vi "barrierOrManMark.vi"(8 "error in (no error)":errorcluster, 9 "Number of Defenders\nWithout Duelist":i32, 10 "Game":refnum<class "Game.lvclass">, 11 "DefendAreaSkill in":refnum<class "DefendAreaSkill.lvclass">) -> (0 "error out":errorcluster, 1 "Enemy position\nto mark":dbl[](array[numeric]), 2 "Type of Defense Barrier":enum16{"Barreira", "Manmark"}(ring), 3 "DefendAreaSkill out":refnum<class "DefendAreaSkill.lvclass">)   [LabVIEW 2024, in "DefendAreaSkill.lvclass"]
uses:
  DefendAreaSkill.lvclass
  Game_class/Game.lvclass
  Team_class/OffensivePlay.ctl
  Game_class/Game.lvclass/Game.ctl
  Team_class/Team.lvclass/Team.ctl
  Events_class/Events.lvclass/Events.ctl
  Object_class/Object.lvclass/Object.ctl
  Object_class/Read x.vi
  Object_class/Read y.vi
  Team_class/Read RobotRef.vi
  Game_class/Read Utilities.lvclass.vi
  Game_class/Read EnemyRef.vi
  Game_class/Read Parameters.lvclass.vi
  Game_class/Read OffensiveTeam.vi
  Game_class/Read BallRef.vi
  Game_class/Read EventsRef.vi
  Events_class/Read id_enemy_ball_possesion.vi
  Team_class/Read OffensivePlay.vi
  Parameters_class/Read AttakingOurselves.vi
  Ally_class/Ally.lvclass
  C:/Users/ROBOIME2/Documents/SSL ROBOIME/SSL_AI/Team_class/Team.lvclass
  Enemy_class/Enemy.lvclass
  Robot_class/Robot.lvclass
  C:/Users/ROBOIME2/Documents/SSL ROBOIME/SSL_AI/Object_class/Object.lvclass
  Utilities_class/Utilities.lvclass
  Parameters_class/Parameters.lvclass
  Ball_class/Ball.lvclass
  Events_class/Events.lvclass
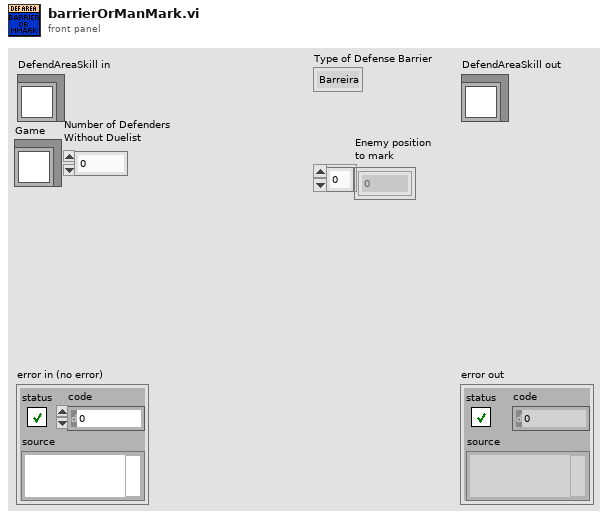
[diagram p1: front panel]
types:
  T1 = typedef "OffensivePlay.ctl" = enum16{"5RobotsPassGamePlay", "5PreparePassGame", "5RobotsKeeperGame", "KeeperPassToStriker", "5RobotsNormalGamePlay", "PrepareKeeperPass", "ACBPass", "ABCPass", "PrepareTriplePass", "TableWithStriker", "TableWith2ndStrikerPlay", "PrepareDoublePass", "PrepareRollToPass", "SimplePass", "PreparePass", "PassToStriker", "BallOutOfField", "PassTo2ndStriker", "StopOffensive", "Prepare Penalty Enemy", "EnemyPossessionAtEnemyField", "EnemyPossesionAtOurField", "TestPlay", "PreparePenaltyAlly", "KickPenaltyAlly", "PrepareKickoffAlly", "PrepareKickoffEnemy", "IndirectEnemy", "DirectEnemy", "PreparePassInGame1", "NormalGame", "DirectKick", "Pass", "Halt", "Timeout", "PassPlay", "PenaltyEnemy"}
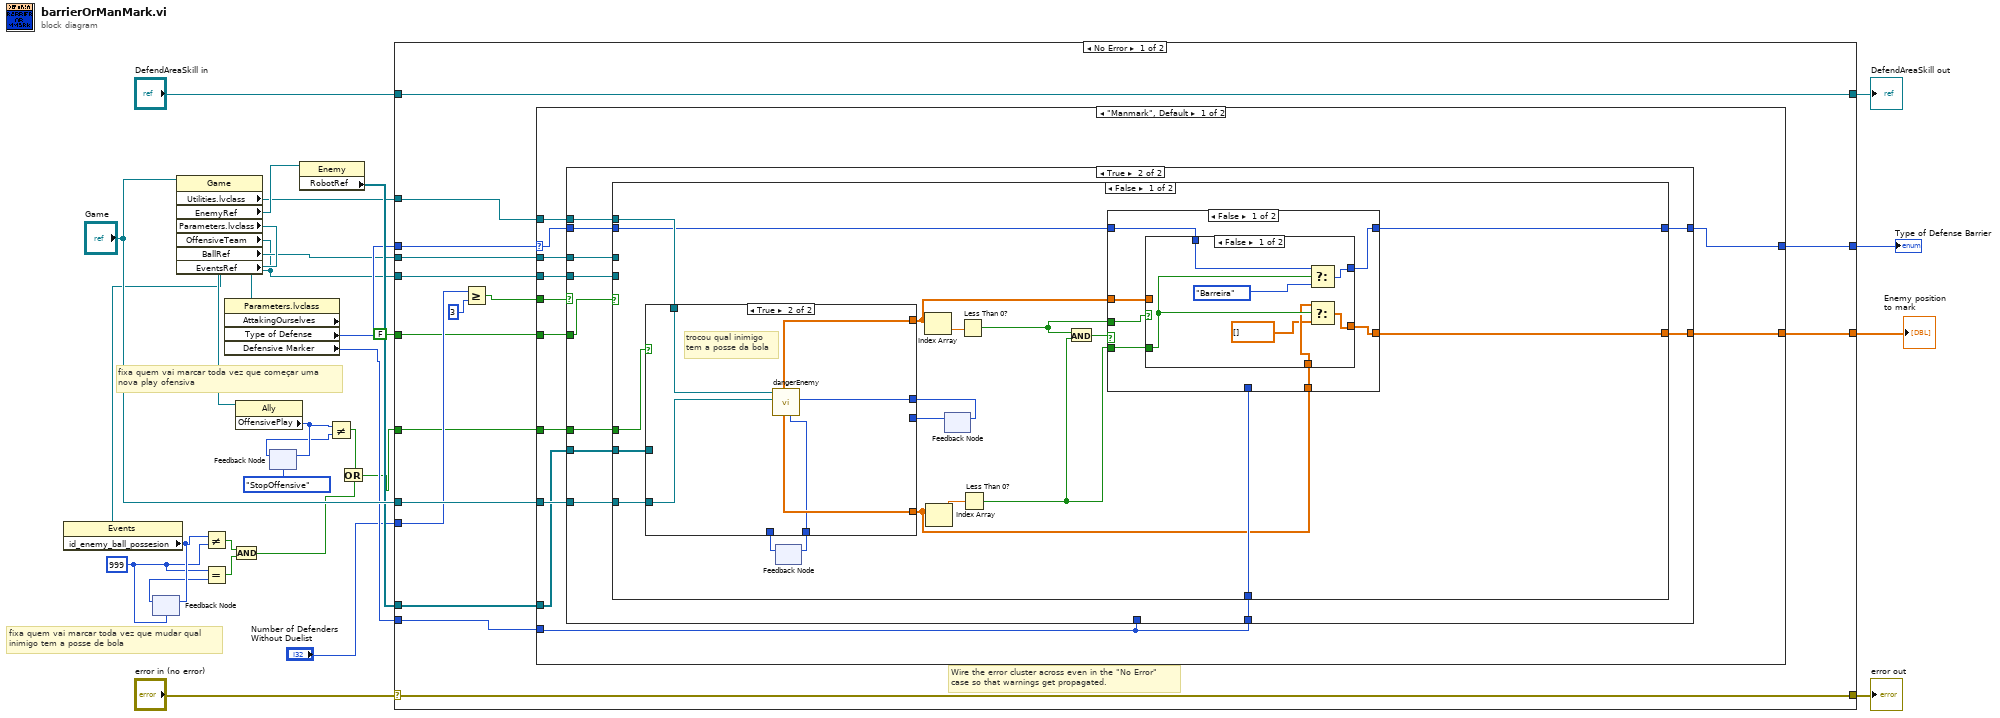
[diagram p0: block diagram]
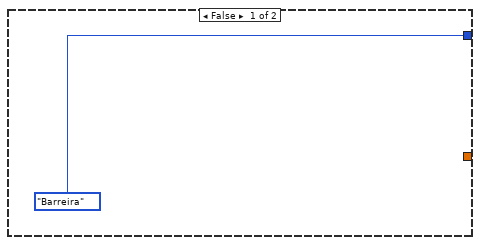
[diagram p2: hidden frame]
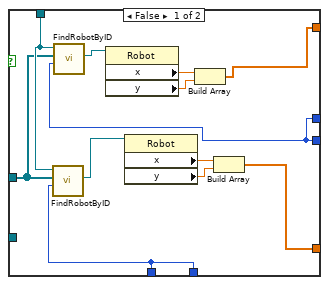
[diagram p3: hidden frame]
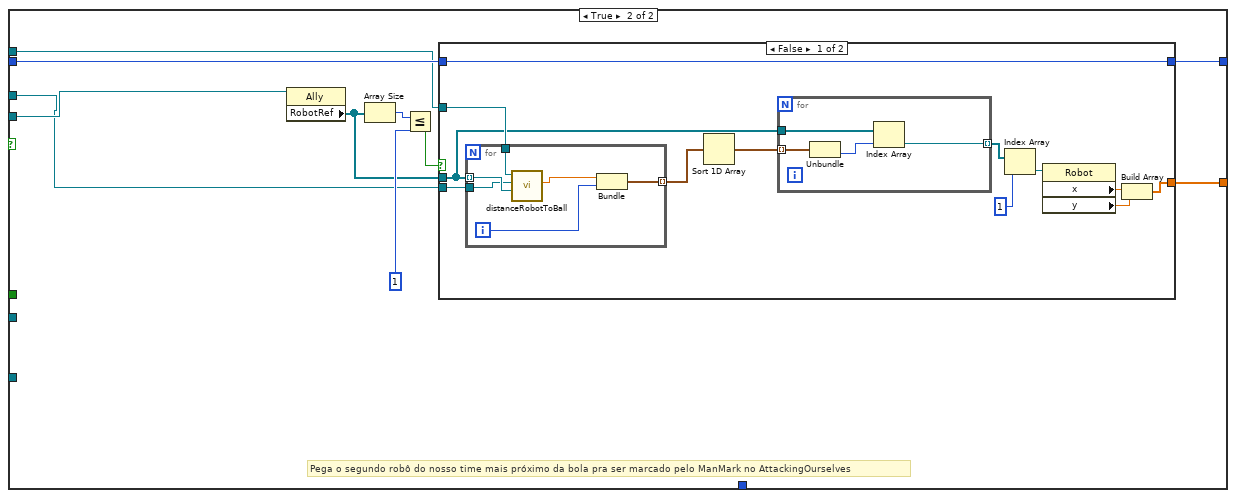
[diagram p7: hidden frame]
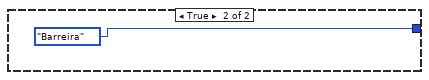
[diagram p8: hidden frame]
diagram:
  w5 = 999
  # "fixa quem vai marcar toda vez que mudar qual\ninimigo tem a posse de bola"
  # "fixa quem vai marcar toda vez que começar uma\nnova play ofensiva"
  n1 = feedback #1(w5) -> (w6:i32)
  n2 = property class="Game"(reference="Game") -> ("Utilities.lvclass"=w16:refnum<class "Utilities.lvclass">, "EnemyRef"=w24:refnum<class "Enemy.lvclass">, "Parameters.lvclass"=w18:refnum<class "Parameters.lvclass">, "OffensiveTeam"=w14:refnum<class "Ally.lvclass">, "BallRef"=w15:refnum<class "Ball.lvclass">, "EventsRef"=w10:refnum<class "Events.lvclass">)  [unwired: 1 in, 2 out]
  n3 = property class="Events"(reference=w10) -> ("id_enemy_ball_possesion"=w7:i32)  [unwired: 1 in, 2 out]
  n4 = feedback-in #1(w7) -> ()
  n5 = Not Equal?(x=w7, y=w5) -> (x != y?=w9:bool)
  n6 = Equal?(x=w5, y=w6) -> (x = y?=w8:bool)
  n7 = property class="Parameters.lvclass" props=["AttakingOurselves", "Type of Defense", "Defensive Marker"](reference=w18) -> ("Type of Defense"=w20:enum16{"Barreira", "Manmark"}, "Defensive Marker"=w21:enum16{"SecondMostDangerous", "MostDangerous"})  [unwired: 1 in, 3 out]
  n8 = And(x=w9, y=w8) -> (x .and. y?=w3:bool)
  n9 = property class="Ally"(reference=w14) -> ("OffensivePlay"=w13:T1)  [unwired: 1 in, 2 out]
  n10 = feedback-in #2(w13) -> ()
  n11 = feedback #2(OffensivePlay."StopOffensive" ("OffensivePlay")) -> (w12:T1)
  n12 = property class="Enemy"(reference=w24) -> ("RobotRef"=w23:refnum<class "Robot.lvclass">[])  [unwired: 1 in, 2 out]
  n13 = Not Equal?(x=w13, y=w12) -> (x != y?=w4:bool)
  n14 = Or(x=w4, y=w3) -> (x .or. y?=w2:bool)
  n15 = case shown="No Error" "error in (no error)" {
    selector: "error in (no error)" -> [w44 w166]
    tunnel: [w44 w166] -> w28
    tunnel: [w45 w165] -> w26
    tunnel: "DefendAreaSkill in" -> [w45 w165]
    tunnel: w20 -> [w43 w164]
    tunnel: [w42 w164] -> w19
    tunnel: "Game" -> [w41 _]
    tunnel: w23 -> [w40 _]
    tunnel: w21 -> [w39 _]
    tunnel: [w38 _] -> w22
    tunnel: "Number of Defenders\nWithout Duelist" -> [w37 _]
    tunnel: FALSE ("AttakingOurselves") -> [w34 _]
    tunnel: w14 -> [w33 _]
    tunnel: w16 -> [w32 _]
    tunnel: w15 -> [w31 _]
    tunnel: w2 -> [w30 _]
    frame No Error {
      # "Wire the error cluster across even in the \"No Error\"\ncase so that warnings get propagated."
      n16 = Greater Or Equal?(x=w37, y=3) -> (x >= y?=w35:bool)
      n17 = case shown="\"Manmark\", Default" w43 {
        selector: w43 -> [w53 w163]
        tunnel: [w56 w163] -> w42
        tunnel: w32 -> [w55 _]
        tunnel: w41 -> [w57 _]
        tunnel: w40 -> [w47 _]
        tunnel: w39 -> [w52 _]
        tunnel: [w54 _] -> w38
        tunnel: w35 -> [w51 _]
        tunnel: w34 -> [w50 _]
        tunnel: w33 -> [w49 _]
        tunnel: w31 -> [w48 _]
        tunnel: w30 -> [w46 _]
        frame "Manmark", Default {
          n18 = case shown="True" w51 {
            tunnel: w57 -> [_ w69]
            tunnel: [enum16{"Barreira", "Manmark"}."Barreira" ("Type of Defense Barrier") w68] -> w56
            tunnel: w52 -> [_ w67]
            tunnel: w55 -> [_ w66]
            tunnel: [_ w65] -> w54
            tunnel: w53 -> [_ w64]
            tunnel: w52 -> [_ _]
            tunnel: w50 -> [_ w63]
            tunnel: w49 -> [_ w62]
            tunnel: w48 -> [_ w61]
            tunnel: w47 -> [_ w60]
            tunnel: w46 -> [_ w59]
            frame False {
            }
            frame True {
              n19 = case shown="False" w63 {
                tunnel: w69 -> [w88 _]
                tunnel: [w84 w135] -> w68
                tunnel: w67 -> [w83 _]
                tunnel: w66 -> [w80 w132]
                tunnel: [w79 w131] -> w65
                tunnel: w64 -> [w76 w134]
                tunnel: w62 -> [_ w139]
                tunnel: w61 -> [_ w130]
                tunnel: w60 -> [w75 _]
                tunnel: w59 -> [w70 _]
                frame False {
                  n20 = feedback #3() -> (w71:i32)  [unwired: 1 in]
                  n21 = feedback #4() -> (w73:u32)  [unwired: 1 in]
                  n22 = case shown="True" w70 {
                    tunnel: w88 -> [_ w106]
                    tunnel: w80 -> [w94 w105]
                    tunnel: [w91 w104] -> w78
                    tunnel: [w89 w103] -> w77
                    tunnel: w75 -> [w93 _]
                    tunnel: [w92 w102] -> w74
                    tunnel: w73 -> [w92 _]
                    tunnel: [w90 w101] -> w72
                    tunnel: w71 -> [w90 _]
                    frame False {
                      n23 = call "FindRobotByID.vi"("id"=w90, "RobotRef"=w93, "Utilities in"=w94) -> ("Robot"=w95:refnum<class "Robot.lvclass">)  [unwired: 5 in, 3 out]
                      n24 = call "FindRobotByID.vi"("id"=w92, "RobotRef"=w93, "Utilities in"=w94) -> ("Robot"=w100:refnum<class "Robot.lvclass">)  [unwired: 5 in, 3 out]
                      n25 = property class="Robot"(reference=w100) -> ("x"=w99:dbl, "y"=w98:dbl)  [unwired: 1 in, 2 out]
                      n26 = property class="Robot"(reference=w95) -> ("x"=w97:dbl, "y"=w96:dbl)  [unwired: 1 in, 2 out]
                      n27 = Build Array(w99, w98) -> (w91:dbl[])
                      n28 = Build Array(w97, w96) -> (w89:dbl[])
                    }
                    frame True {
                      # "trocou qual inimigo\ntem a posse da bola"
                      n29 = call "dangerEnemy.vi"("Game"=w106, "Utilities in"=w105) -> ("Id do Inimigo Mais Próximo"=w102:u32, "id do segundo inimigo mais perigoso"=w101:i32, "Pos do segundo inimigo\nperigoso"=w103:dbl[], "Pos do inimigo\nmais perigoso"=w104:dbl[])  [unwired: 3 in, 3 out]
                    }
                  }
                  n30 = feedback-in #3(w72) -> ()
                  n31 = Index Array(array=w78) -> (element=w87:dbl)  [unwired: 1 in]
                  n32 = Index Array(array=w77) -> (element=w86:dbl)  [unwired: 1 in]
                  n33 = feedback-in #4(w74) -> ()
                  n34 = Less Than 0?(x=w87) -> (x < 0?=w82:bool)
                  n35 = Less Than 0?(x=w86) -> (x < 0?=w81:bool)
                  n36 = And(x=w82, y=w81) -> (x .and. y?=w85:bool)
                  n37 = case shown="False" w85 {
                    tunnel: [w112 w123] -> w84
                    tunnel: w83 -> [_ w127]
                    tunnel: w82 -> [w113 _]
                    tunnel: w81 -> [w111 _]
                    tunnel: [w110 w126] -> w79
                    tunnel: w78 -> [w109 w125]
                    tunnel: w77 -> [w108 w124]
                    tunnel: w76 -> [w107 w123]
                    frame False {
                      n38 = case shown="False" w113 {
                        tunnel: [w118 w121] -> w112
                        tunnel: w111 -> [w120 _]
                        tunnel: [w116 w122] -> w110
                        tunnel: w109 -> [_ w122]
                        tunnel: w108 -> [w117 _]
                        tunnel: w107 -> [w119 w121]
                        frame False {
                          n39 = Select(t=w119, s=w120, f=enum16{"Barreira", "Manmark"}."Barreira" ("Type of Defense Barrier")) -> (s? t:f=w118:enum16{"Barreira", "Manmark"})
                          n40 = Select(t=w117, s=w120, f=dbl[] []) -> (s? t:f=w116:dbl[])
                        }
                        frame True {
                          # "Just dangerous is in our side"
                        }
                      }
                    }
                    frame True {
                      # "Both dangerous\nand second dangerous\nare in our side"
                      n41 = case shown="\"MostDangerous\", Default" w127 {
                        tunnel: [w128 w129] -> w126
                        tunnel: w125 -> [_ w129]
                        tunnel: w124 -> [w128 _]
                        frame "SecondMostDangerous" {
                        }
                        frame "MostDangerous", Default {
                        }
                      }
                    }
                  }
                }
                frame True {
                  # "Pega o segundo robô do nosso time mais próximo da bola pra ser marcado pelo ManMark no AttackingOurselves"
                  n42 = property class="Ally"(reference=w139) -> ("RobotRef"=w133:refnum<class "Robot.lvclass">[])  [unwired: 1 in, 2 out]
                  n43 = Array Size(array=w133) -> (size(s)=w138:i32)
                  n44 = Less Or Equal?(x=w138, y=1) -> (x <= y?=w136:bool)
                  n45 = case shown="False" w136 {
                    tunnel: [w151 enum16{"Barreira", "Manmark"}."Barreira" ("Type of Defense Barrier")] -> w135
                    tunnel: w134 -> [w151 _]
                    tunnel: w133 -> [w147 _]
                    tunnel: w132 -> [w148 _]
                    tunnel: [w141 _] -> w131
                    tunnel: w130 -> [w140 _]
                    frame False {
                      n46 = for {
                        tunnel: w147 -> [w158] mode=indexing
                        tunnel: [w160] -> w149 mode=indexing
                        tunnel: w148 -> [w159]
                        tunnel: w140 -> [w156]
                        i -> [w161]
                        n47 = call "distanceRobotToBall.vi"("Robot"=w158, "Ball"=w156, "Utilities in"=w159) -> ("Distance Robot To Ball"=w157:dbl)  [unwired: 6 in, 2 out]
                        n48 = Bundle("Distance Robot To Ball"=w157, w161) -> (w160:cluster{"Distance Robot To Ball":dbl, i32})  [unwired: 1 in]
                      }
                      n49 = Sort 1D Array(array=w149) -> (sorted array=w150:cluster{"Distance Robot To Ball":dbl, i32}[])
                      n50 = for {
                        tunnel: w150 -> [w154] mode=indexing
                        tunnel: w147 -> [w155]
                        tunnel: [w152] -> w146 mode=indexing
                        n51 = Unbundle(w154) -> (w153:i32)  [unwired: 1 out]
                        n52 = Index Array(array=w155, index=w153) -> (element=w152:refnum<class "Robot.lvclass">)
                      }
                      n53 = Index Array(array=w146, index=1) -> (element=w144:refnum<class "Robot.lvclass">)
                      n54 = property class="Robot"(reference=w144) -> ("x"=w143:dbl, "y"=w142:dbl)  [unwired: 1 in, 2 out]
                      n55 = Build Array(w143, w142) -> (w141:dbl[])
                    }
                    frame True {
                    }
                  }
                }
              }
            }
          }
        }
        frame "Barreira" {
        }
      }
    }
    frame Error {
    }
  }
  "error out" <- w28
  "DefendAreaSkill out" <- w26
  "Enemy position\nto mark" <- w22
  "Type of Defense Barrier" <- w19
